vi "Command and read pump.vi"(8 "error in (no error)":errorcluster, 9 "command":string, 10 "Address (00)":i32, 11 "VISA resource name":refnum<visa-resource-name>) -> (0 "error out":errorcluster, 1 "Output String":string, 2 "Pump status":T2 items=["Error - Can't read status"=-1, "Stopped"=0, "Infusing"=1, "Withdrawing"=2, "Pump stalled"=3, "Stopped at infuse limit"=4, "Stopped at withdraw limit"=5, "Emergency stop"=6, "Stopped at target volume"=7], 3 "VISA resource name out":refnum<visa-resource-name>, 4 "Numeric result":dbl, 5 "String result":string)   [LabVIEW 2015]
doc: "This VI sends a specificed commnd to the pump and returns the pump response and status.\n\nModified from original which is Copyright 2005, National Instruments Corporation.\n\nModifications Copyright 2009, Jeff Gelles, Brandeis University"
uses:
  Pump status.ctl
panel:
  in  "Log":enum16{"None", "All", "Error only"}(ring)
  in  "Log":T1(array[cluster])
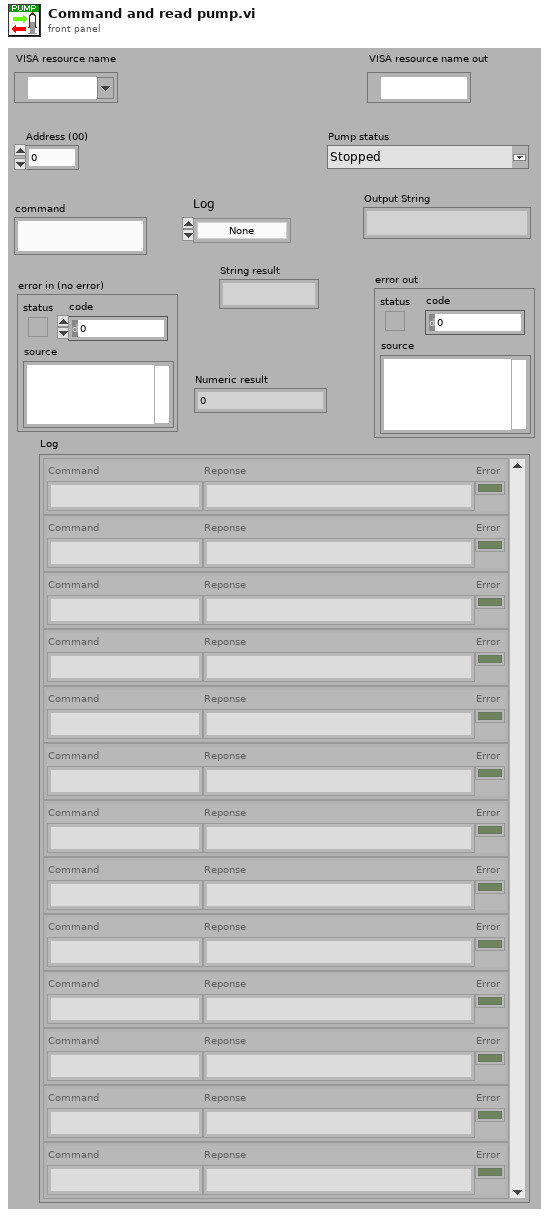
[diagram p1: front panel]
types:
  T1 = cluster{"Command":string, "Reponse":string, "Error":bool}[]
  T2 = typedef "Pump status.ctl" = i8
  T3 = cluster{string, "Output String":string, "status":bool}
  T4 = cluster{"Command":string, "Output String":string, "status":bool}[]
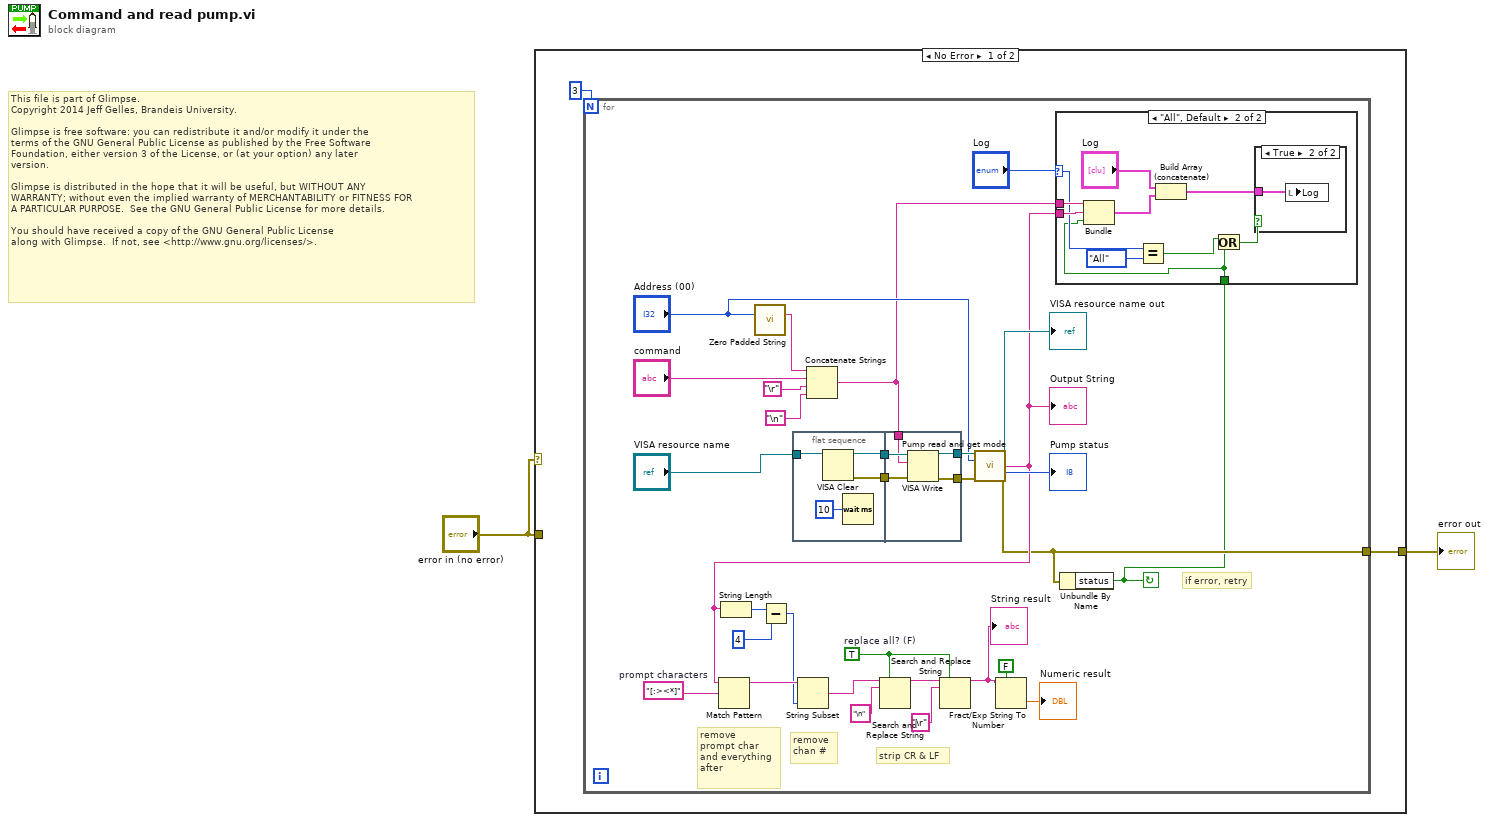
[diagram p0: block diagram]
diagram:
  # "This file is part of Glimpse. \nCopyright 2014 Jeff Gelles, Brandeis University.    \n\nGlimpse is free software: you can redistribute it and/or modify it under the \nterms of the GNU General Public License as published by the Free Software \nFoundation, either version 3 of the License, or (at your option) any later \nversion.\n\nGlimpse is distributed in the hope that it will be useful, but WITHOUT ANY \nWARRANTY; without even the implied warranty of MERCHANTABILITY or FITNESS FOR \nA PARTICULAR PURPOSE.  See the GNU General Public License for more details.\n\nYou should have received a copy of the GNU General Public License\nalong with Glimpse.  If not, see <http://www.gnu.org/licenses/>."
  n1 = case shown="No Error" "error in (no error)" {
    tunnel: [w4 w55] -> w2
    tunnel: "error in (no error)" -> [_ w55]
    frame No Error {
      n2 = for {
        N: 3 -> [_]
        tunnel: [w11] -> w4
        stop <- w9 continue-if-true
        w8 = TRUE  # replace all? (F)
        w26 = "[:><*]"  # prompt characters
        # "if error, retry"
        # "strip CR & LF"
        # "remove \nchan #"
        # "remove \nprompt char\nand everything\nafter"
        n3 = call "Zero Padded String.vi"("Address (00)"="Address (00)") -> ("Zero Padded Address String"=w27:string)  [unwired: 14 out]
        n4 = flat-sequence {
          tunnel: "VISA resource name" -> [w48]
          tunnel: [w47] -> w34
          tunnel: [w46] -> w5
          tunnel: [w54] -> w30
          tunnel: [w53] -> w29
          tunnel: w6 -> [w51]
          tunnel: w34 -> [w52]
          tunnel: w5 -> [w50]
          frame #0 {
            n5 = VISA Clear(VISA resource name=w48) -> (VISA resource name out=w47:refnum<visa-resource-name>, error out=w46:errorcluster)  [unwired: 1 in]
            n6 = Wait (ms)(milliseconds to wait=u32 10) -> ()  [unwired: 1 out]
          }
          frame #1 {
            n7 = VISA Write(VISA resource name=w52, write buffer=w51, error in (no error)=w50) -> (VISA resource name out=w54:refnum<visa-resource-name>, error out=w53:errorcluster)  [unwired: 1 out]
          }
        }
        n8 = Concatenate Strings(w27, "command", "\r", "\n") -> (w6:string)
        n9 = call "Pump read and get mode.vi"("VISA resource name"=w30, "Address (00)"="Address (00)", "error in (no error)"=w29) -> ("VISA resource name out"=→"VISA resource name out":refnum<visa-resource-name>, "Output String"=w13:string, "Pump status"=→"Pump status":T2, "error out"=w11:errorcluster)  [unwired: 9 out]
        "Output String" <- w13
        n10 = Match Pattern(string=w13, regular expression=w26) -> (before substring=w25:string)  [unwired: 4 out]
        n11 = String Length(string=w13) -> (length=w24:i32)
        n12 = Subtract(x=w24, y=4) -> (x-y=w22:i32)
        n13 = String Subset(string=w25, length (rest)=w22) -> (substring=w21:string)  [unwired: 1 out]
        n14 = Search and Replace String(replace all?=w8, input string=w21, search string="\n") -> (result string=w18:string)  [unwired: 1 in, 7 out]
        n15 = Search and Replace String(replace all?=w8, input string=w18, search string="\r") -> (result string=w15:string)  [unwired: 1 in, 7 out]
        "String result" <- w15
        n16 = Fract/Exp String To Number(use system decimal point (T)=FALSE, string=w15) -> (number=→"Numeric result":dbl)  [unwired: 3 out]
        n17 = Unbundle By Name(w11) -> ("status"=w9:bool)
        n18 = case shown="\"All\", Default" "Log" {
          selector: "Log" -> [_ w37]
          tunnel: w6 -> [_ w44]
          tunnel: w13 -> [_ w43]
          tunnel: w9 -> [_ w35]
          frame "None" {
          }
          frame "All", Default {
            n19 = Bundle(w44, "Output String"=w43, "status"=w35) -> (w41:T3)  [unwired: 1 out]
            n20 = Equal?(x=w37, y=enum16{"None", "All", "Error only"}."All") -> (x = y?=w38:bool)
            n21 = Build Array (concatenate)("Log", w41) -> (w40:T4)
            n22 = Or(x=w38, y=w35) -> (x .or. y?=w39:bool)
            n23 = case shown="True" w39 {
              tunnel: w40 -> [_ w45]
              frame False {
              }
              frame True {
                n24 = local write "Log"(w45) -> ()
              }
            }
          }
        }
      }
    }
    frame Error {
    }
  }
  "error out" <- w2
